vi "DrawWinScreen.vi"(8 "error in (no error)":errorcluster, 11 "Snake in":refnum<class "SnakeGame.lvclass">) -> (0 "error out":errorcluster, 3 "Snake out":refnum<class "SnakeGame.lvclass">)   [LabVIEW 2019, in "RT_Game.lvlib" / "SnakeGame.lvclass"]
uses:
  SnakeGame.lvclass
  C:/Users/FreshBob/Dropbox/VIs/myRIO_GameConsole/RT/RT_Game/Game/Game.lvclass
  SnakeGame.lvclass/SnakeGame.ctl
  Game/Coordinate.ctl
  Snake/Snake.lvclass/Snake.ctl
  Snake/Read Color.vi
  Snake/Read Length.vi
  Game/Game.lvclass
  Snake/Snake.lvclass
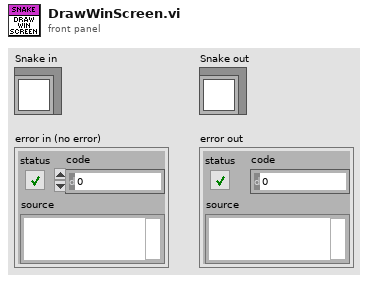
[diagram p1: front panel]
types:
  T1 = typedef "RT_Game.lvlib/Game.lvclass/Coordinate.ctl" = cluster{"x":dbl, "y":dbl}
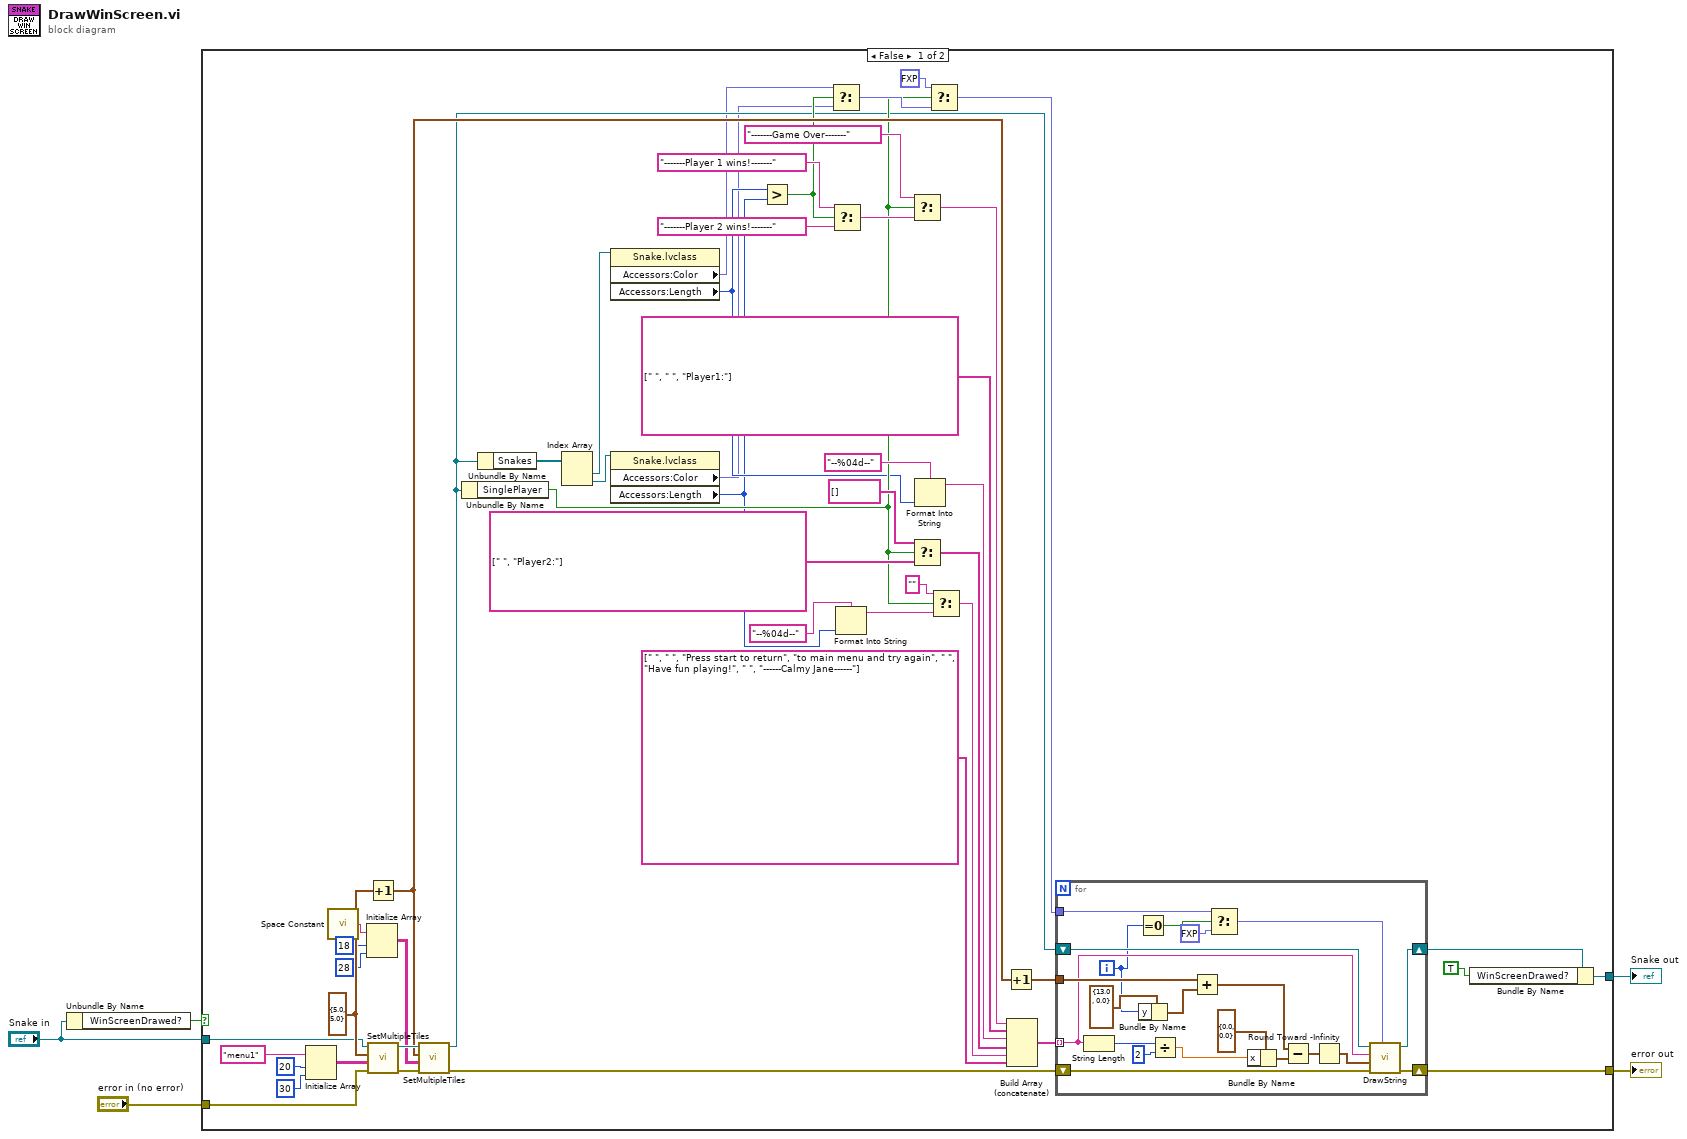
[diagram p0: block diagram]
diagram:
  n1 = Unbundle By Name("Snake in") -> ("WinScreenDrawed?"=w1:bool)
  n2 = case shown="False" w1 {
    tunnel: "Snake in" -> [w14 w78]
    tunnel: "error in (no error)" -> [w54 w77]
    tunnel: [w42 w77] -> w4
    tunnel: [w16 w78] -> w3
    frame False {
      w47 = T1 {"x"=5.0, "y"=5.0} ("Position")
      n3 = Initialize Array("menu1" ("element"), 20 ("dimension size"), 30 ("dimension size")) -> (w51:string[][])
      n4 = call <vilib>:"Space Constant.vi"() -> ("String"=w46:string)
      n5 = Initialize Array(w46, 18 ("dimension size"), 28 ("dimension size")) -> (w43:string[][])
      n6 = Increment(x=w47) -> (x+1=w38:T1)
      n7 = call "SetMultipleTiles.vi"("error in (no error)"=w54, "TileCodes"=w51, "Position"=w47, "Game in"=w14) -> ("error out"=w55:errorcluster, "Game out"=w48:refnum<class "SnakeGame.lvclass">)  [unwired: 6 in]
      n8 = call "SetMultipleTiles.vi"("error in (no error)"=w55, "TileCodes"=w43, "Position"=w38, "Game in"=w48) -> ("error out"=w49:errorcluster, "Game out"=w13:refnum<class "SnakeGame.lvclass">)  [unwired: 6 in]
      n9 = Unbundle By Name(w13) -> ("SinglePlayer"=w17:bool)
      n10 = Unbundle By Name(w13) -> ("Snakes"=w12:refnum<class "Snake.lvclass">[])
      n11 = Index Array(array=w12) -> (element #1=w11:refnum<class "Snake.lvclass">, element #2=w8:refnum<class "Snake.lvclass">)  [unwired: 2 in]
      n12 = property class="Snake.lvclass"(reference=w11) -> ("Accessors:Color"=w10:fxp<+,3,3>, "Accessors:Length"=w9:i16)  [unwired: 1 in, 2 out]
      n13 = property class="Snake.lvclass"(reference=w8) -> ("Accessors:Color"=w7:fxp<+,3,3>, "Accessors:Length"=w6:i16)  [unwired: 1 in, 2 out]
      n14 = Greater?(x=w9, y=w6) -> (0:w29:bool)
      n15 = Select(t=w10, s=w29, f=w7) -> (s? t:f=w28:fxp<+,3,3>)
      n16 = Select(t="-------Player 1 wins!-------" ("element"), s=w29, f="-------Player 2 wins!-------" ("element")) -> (s? t:f=w26:string)
      n17 = Format Into String(format string="--%04d--", w6) -> (resulting string=w33:string)  [unwired: 2 in, 1 out]
      n18 = Select(t="-------Game Over-------" ("element"), s=w17, f=w26) -> (s? t:f=w27:string)
      n19 = Select(t=string[] [], s=w17, f=string[] [" ", "Player2:"] ("element")) -> (s? t:f=w22:string[])
      n20 = Format Into String(format string="--%04d--", w9) -> (resulting string=w36:string)  [unwired: 2 in, 1 out]
      n21 = Select(t=fxp<+,3,3> 0.0, s=w17, f=w28) -> (s? t:f=w24:fxp<+,3,3>)
      n22 = Select(t="" ("f"), s=w17, f=w33) -> (s? t:f=w19:string)
      n23 = Increment(x=w38) -> (x+1=w37:T1)
      n24 = Build Array (concatenate)(w27, string[] [" ", " ", "Player1:"] ("element"), w36, w22, w19, string[] [" ", " ", "Press start to return", "to main menu and try again", " ", "Have fun playing!", " ", "------Calmy Jane------"] ("element")) -> (w39:string[])
      n25 = for {
        shift-right: [w75] -> w42
        shift-left: w49 -> [w76]
        shift-right: [w74] -> w41
        shift-left: w13 -> [w73]
        tunnel: w39 -> [w67] mode=indexing
        tunnel: w37 -> [w72]
        tunnel: w24 -> [w57]
        i -> [w59]
        n26 = String Length(string=w67) -> (length=w68:i32)
        n27 = Equal To 0?(x=w59) -> (x = 0?=w58:bool)
        n28 = Bundle By Name(cluster=T1 {"x"=13.0, "y"=0.0} ("y"), "y"=w59) -> (w64:T1)
        n29 = Divide(x=w68, y=2) -> (x/y=w63:dbl)
        n30 = Add(x=w72, y=w64) -> (x+y=w70:T1)
        n31 = Select(t=w57, s=w58, f=fxp<+,3,3> 7.0 ("Color (7=white)")) -> (s? t:f=w60:fxp<+,3,3>)
        n32 = Bundle By Name(cluster=T1 {"x"=0.0, "y"=0.0} ("y"), "x"=w63) -> (w66:T1)
        n33 = Subtract(x=w70, y=w66) -> (x-y=w65:T1)
        n34 = Round Toward -Infinity(1:w65) -> (0:w56:T1)
        n35 = call "DrawString.vi"("Color (7=white)"=w60, "error in (no error)"=w76, "Coordinate"=w56, "String"=w67, "RT_Game.lvlib:Game.lvclass"=w73) -> ("error out"=w75:errorcluster, "RT_Game.lvlib:Game.lvclass 2"=w74:refnum<class "SnakeGame.lvclass">)  [unwired: 5 in]
      }
      n36 = Bundle By Name(cluster=w41, "WinScreenDrawed?"=TRUE) -> (w16:refnum<class "SnakeGame.lvclass">)
    }
    frame True {
    }
  }
  "Snake out" <- w3
  "error out" <- w4
